vi "32[1]-Trace Data Collection.vi"(8 "error in (no error)":errorcluster, 11 "Terminate TRID":u32) -> (0 "error out":errorcluster)   [LabVIEW 2020, in "SECS Scenarios.lvlib" / "Scenarios Class.lvclass"]
uses:
  Scenarios Class.lvclass
  32[1]-Trace Data Collection.ctl
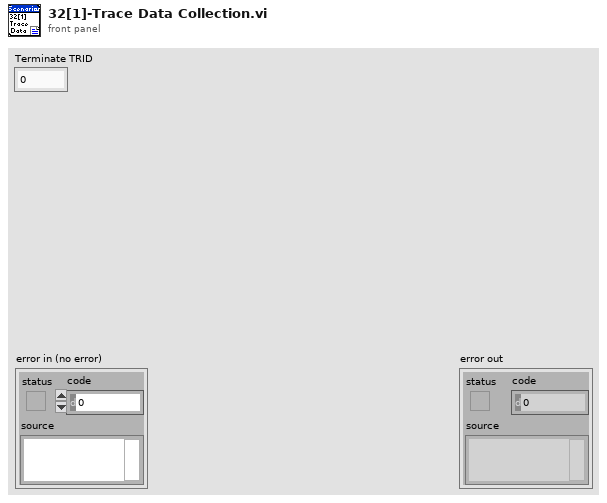
[diagram p1: front panel]
types:
  T1 = typedef "SECS Scenarios.lvlib/Scenarios Class.lvclass/32[1]-Trace Data Collection.ctl" = cluster{"Terminate TRID":u32}
  T2 = typedef "SECS Scenarios.lvlib/Scenarios Class.lvclass/Broadcast Refnum.ctl" = cluster{"13-EnableDisable Alarm":refnum<user-event>, "15-Process Program Request":refnum<user-event>, "16-Process Program Send":refnum<user-event>, "17-Deleting a Process Program by Host":refnum<user-event>, "18-Host Requests Equipment Process Program Directory":refnum<user-event>, "19-Equipment Process Program Uploading":refnum<user-event>, "20[1]-Process Program Downloading":refnum<user-event>, "20[2]-Process Program Downloading":refnum<user-event>, "22-Host Sends Information to Equipment":refnum<user-event>, "26-Host Requests to Enter OFF-Line":refnum<user-event>, "27-Host Requests to Enter On-Line":refnum<user-event>, "28[1]-Remote Control[PP-SELECT]":refnum<user-event>, "28[2]-Remote Control[START]":refnum<user-event>, "28[3]-Remote Control[STOP]":refnum<user-event>, "28[4]-Remote Control[LOCAL]":refnum<user-event>, "28[5]-Remote Control[REMOTE]":refnum<user-event>, "28[6]-Remote Control[RCMD]":refnum<user-event>, "30-Host Requests Equipment to Set Time":refnum<user-event>, "31-Host Requests Time Value from Equipment":refnum<user-event>, "32[1]-Trace Data Collection":refnum<user-event>, "32[2]-Trace Data Collection":refnum<user-event>}
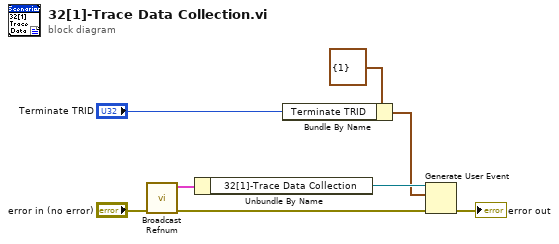
[diagram p0: block diagram]
diagram:
  n1 = call "Broadcast Refnum.vi"("error in"="error in (no error)") -> ("error out"=w7:errorcluster, "Broadcast Refnum"=w8:T2)  [unwired: 9 in]
  n2 = Unbundle By Name(w8) -> ("32[1]-Trace Data Collection"=w6:refnum<user-event>)
  n3 = Bundle By Name(cluster=T1 {"Terminate TRID"=1} ("32[1]-Trace Data Collection"), "Terminate TRID"="Terminate TRID") -> (w2:T1)
  n4 = Generate User Event(user event=w6, event data cluster=w2, error in=w7) -> (error out=→"error out":errorcluster)  [unwired: 1 in, 1 out]
